vi "MCLB.vi"(11 "Error_In":errorcluster) -> (4 "Multicolumn_Listbox":i32[](listbox), 15 "Errror_Out":errorcluster)   [LabVIEW 2023]
uses:
  Controls/Names_Box.ctl
  <vilib>/Utility/miscctls.llb/LVPositionTypeDef.ctl
panel:
  in  "Names_Box":T1
  # "Solins List and Track"
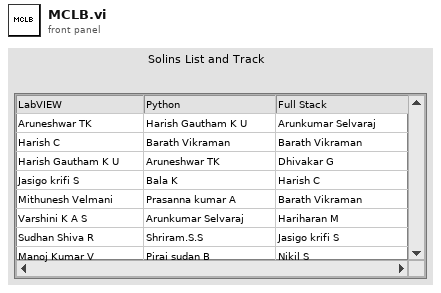
[diagram p1: front panel]
types:
  T1 = typedef "Names_Box.ctl" = string
  T2 = typedef "LVPositionTypeDef.ctl" = cluster{"Left":i32, "Top":i32}
  T3 = typedef "LVPoint32TypeDef.ctl" = cluster{"Horizontal":i32, "Vertical":i32}
  T4 = typedef "LVRowAndColumnTypeDef.ctl" = cluster{"Row":i32, "Column":i32}
  T5 = enum16{"Left Button", "Center Button", "Right Button", "Window Close"}
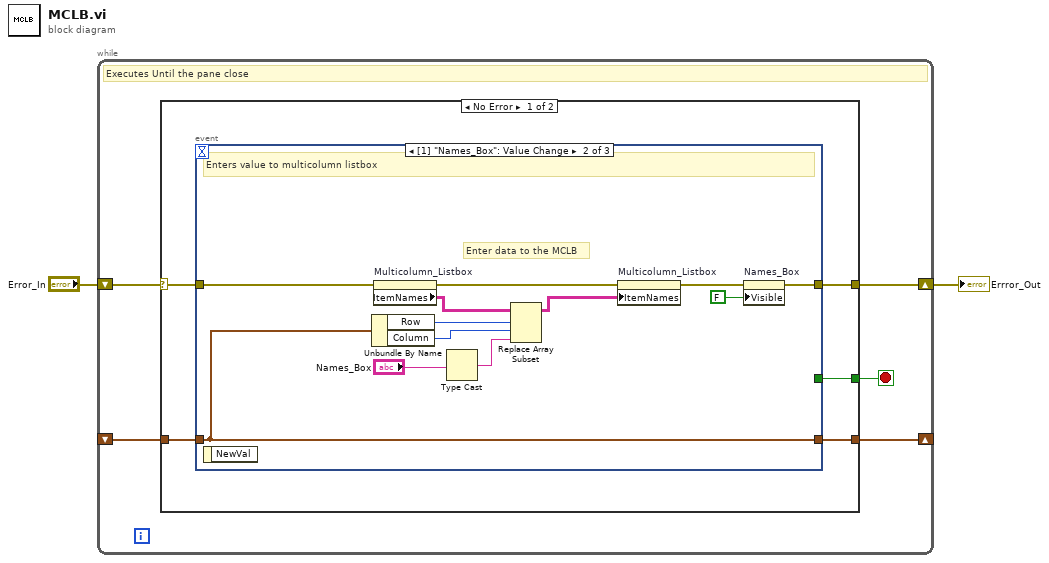
[diagram p0: block diagram]
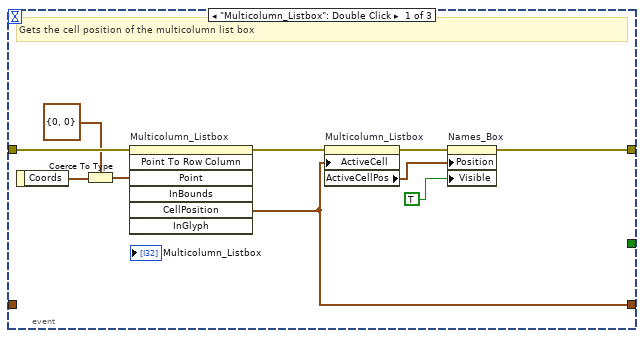
[diagram p2: hidden frame]
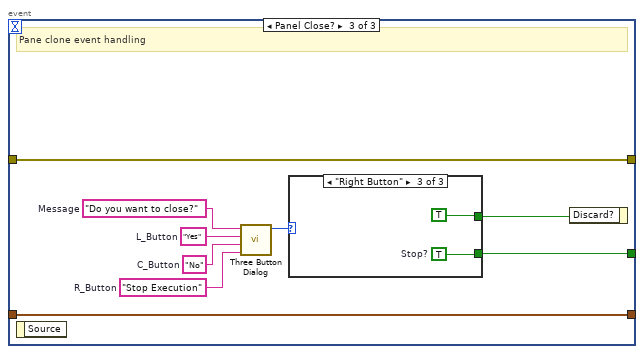
[diagram p3: hidden frame]
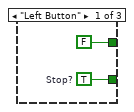
[diagram p4: hidden frame]
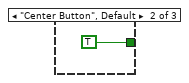
[diagram p5: hidden frame]
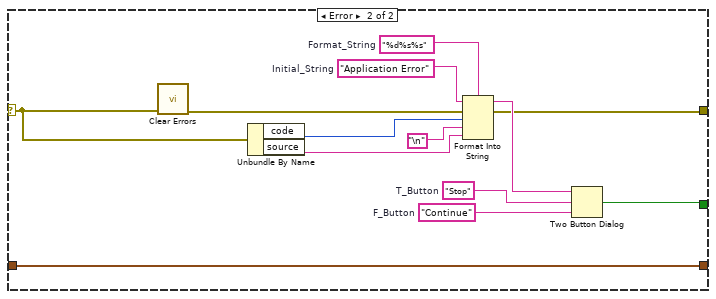
[diagram p6: hidden frame]
diagram:
  n1 = while {
    shift-right: [w6] -> _
    shift-left: _ -> [w7]
    shift-right: [w3] -> w1
    shift-left: "Error_In" -> [w4]
    stop <- w5 stop-if-true
    # "Executes Until the pane close"
    n2 = case shown="No Error" w4 {
      selector: w4 -> [w9 w52]
      tunnel: w7 -> [w12 w50]
      tunnel: [w11 w50] -> w6
      tunnel: [w10 w49] -> w5
      tunnel: [w8 w51] -> w3
      frame No Error {
        n3 = event shown="[1] \"Names_Box\": Value Change" {
          selector: _ -> [_ _ _]
          dyn-events: _ -> [_ _ _]
          timeout: _ -> [_ _ _]
          tunnel: w12 -> [_ w31 w43]
          tunnel: [w21 w31 w43] -> w11
          tunnel: [_ _ w36] -> w10
          tunnel: w9 -> [w19 w29 w35]
          tunnel: [w16 w24 w35] -> w8
          event "Multicolumn_Listbox": Double Click {
            # "Gets the cell position of the multicolumn list box"
            n4 = event-data() -> ("Coords"=w15:T3)  [unwired: 1 in]
            n5 = Coerce To Type(0:w15, 1:T2 {"Left"=0, "Top"=0} ("Point")) -> (2:w13:T2)
            n6 = invoke on="Multicolumn_Listbox" class="MCListbox (strict)" method="Point To Row Column"(error in=w19, "Point"=w13) -> (error out=w18:errorcluster, "CellPosition"=w21:T4)  [unwired: 5 in, 5 out]
            n7 = property on="Multicolumn_Listbox" class="MCListbox (strict)"(error in=w18, "ActiveCell"=w21) -> (error out=w17:errorcluster, "ActiveCellPos"=w22:T2)  [unwired: 1 in, 1 out]
            n8 = property on="Names_Box" class="CmbBox (strict)"(error in=w17, "Position"=w22, "Visible"=TRUE) -> (error out=w16:errorcluster)  [unwired: 1 in, 1 out]
          }
          event Value Change {
            # "Enter data to the MCLB"
            # "Enters value to multicolumn listbox"
            n9 = event-data() -> ()  [unwired: 1 in, 1 out]
            n10 = Unbundle By Name(w31) -> ("Row"=w32:i32, "Column"=w33:i32)
            n11 = property on="Multicolumn_Listbox" class="MCListbox (strict)"(error in=w29) -> (error out=w28:errorcluster, "ItemNames"=w30:string[][])  [unwired: 1 in, 1 out]
            n12 = Type Cast(x="Names_Box") -> (*(type *) &x=w26:string)  [unwired: 1 in]
            n13 = Replace Array Subset(array=w30, new element=w26, index (row)=w32, index (col)=w33) -> (w34:string[][])
            n14 = property on="Multicolumn_Listbox" class="MCListbox (strict)"(error in=w28, "ItemNames"=w34) -> (error out=w25:errorcluster)  [unwired: 1 in, 1 out]
            n15 = property on="Names_Box" class="CmbBox (strict)"(error in=w25, "Visible"=FALSE) -> (error out=w24:errorcluster)  [unwired: 1 in, 1 out]
          }
          event Panel Close? {
            w39 = "Stop Execution"  # R_Button
            w40 = "No"  # C_Button
            w41 = "Yes"  # L_Button
            w42 = "Do you want to close?"  # Message
            # "Pane clone event handling"
            n16 = event-data() -> ()  [unwired: 1 in, 1 out]
            n17 = call <vilib>:"Three Button Dialog.vi"("Right Button Text (\"Cancel\")"=w39, "Center Button Text (\"No\")"=w40, "Left Button Text (\"Yes\")"=w41, "message"=w42) -> ("Which Button?"=w38:T5)  [unwired: 7 in]
            n18 = case shown="\"Right Button\"" w38 {
              tunnel: [FALSE TRUE TRUE] -> w37
              tunnel: [w44 _ w48] -> w36
              frame "Left Button" {
                w44 = TRUE  # Stop?
              }
              frame "Center Button", Default {
              }
              frame "Right Button" {
                w48 = TRUE  # Stop?
              }
            }
            n19 = event-data("Discard?"=w37) -> ()  [unwired: 1 in, 1 out]
          }
        }
      }
      frame Error {
        w54 = "%d%s%s"  # Format_String
        w55 = "Application Error"  # Initial_String
        w56 = "Stop"  # T_Button
        w57 = "Continue"  # F_Button
        n20 = call <vilib>:"Clear Errors.vi"("error in (no error)"=w52) -> ("error out"=w59:errorcluster)  [unwired: 5 in, 1 out]
        n21 = Unbundle By Name(w52) -> ("code"=w61:i32, "source"=w60:string)
        n22 = Format Into String(format string=w54, initial string=w55, error in=w59, w61, "\n", w60) -> (resulting string=w58:string, error out=w51:errorcluster)
        n23 = Two Button Dialog(message=w58, 1:w57, 2:w56) -> (T button?=w49:bool)
      }
    }
  }
  "Errror_Out" <- w1
